vi "Stoerungen (385-448) - VFS4.vi"(8 "Fehler (Eingang)":errorcluster caption="Fehler (Eingang, kein Fehler)") -> (0 "Fehler (Ausgang)":errorcluster, 3 "Störungen 385-448":u64)   [LabVIEW 2015]
uses:
  PNS/Parameternamen PNS.ctl
  PNS/PNS.lvlib
  Stoerungen.lvlib
  Stoerungen Messgeraet/Aktionen Kommunikation Stoerung.ctl
  Seiten/System Einstellungen/System Einstellungen.lvlib
  Seiten/System Einstellungen/Aktioen FGV System.ctl
  PNS/Aktionen FGV Istwerte.ctl
  cRIO/Stoermeldungen/Stoerungen 385-448.ctl
  cRIO/Stoermeldungen/Stoermeldungen.lvlib
panel:
  # "Störmeldungen PNS (385-448)"
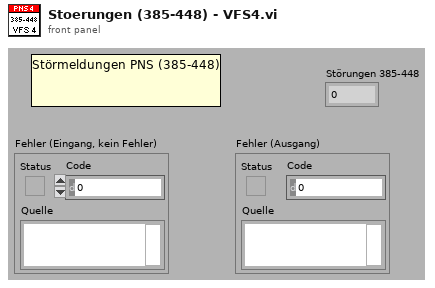
[diagram p1: front panel]
types:
  T1 = typedef "System Einstellungen.lvlib/Aktioen FGV System.ctl" = enum16{"lesen", "laden", "speichern", "Optionen schreiben", "Zeitstempel", "Reset BMP", "Reset SQP", "Wartung"}
  T2 = typedef "System Einstellungen.lvlib/Optionen.ctl" = cluster{"Störmeldep.":bool, "Betriebszustände":bool, "LN2 Befüllung":bool, "Klimaanlage ?":bool, "AK in ppm":bool, "log Cal-Gas":bool, "log 0-Gas":bool, "log CG zu PNS":bool, "Reserve":bool, "Reserve1":bool, "PNS?":bool, "Container":bool, "Mit N2 spülen":bool, "Span Gas Auswahl":T3, "VFS 1":bool, "VFS 2":bool, "VFS 3":bool, "VFS 4":bool, "TRE08":bool, "Leakcheck vor Kal":bool, "Amium 10-Fach":bool}
  T3 = typedef "Funktionstasten.lvlib/Spaneingang.ctl" = u16
  T4 = typedef "PNS.lvlib/Parameternamen PNS.ctl" = enum16{"Heizkreis 1", "Heizkreis 2", "Heizkreis 3", "Heizkreis 4", "Heizkreis 5", "Heizkreis 6", "Heizkreis 7", "Heizkreis 8"}
  T5 = typedef "PNS.lvlib/Aktionen FGV Istwerte.ctl" = enum16{"lesen", "initialisieren", "schreiben", "Störungen"}
  T6 = typedef "Stoerungen.lvlib/Aktionen Kommunikation Stoerung.ctl" = enum16{"lesen", "init", "FT-IR Komm", "FT-IR Betriebsart", "FT-IR Hintergrund", "cRIO Komm", "PNS Komm", "Dichtheitstest", "Life Bit", "FTIR Komm AK", "PMA Komm", "FID Komm", "PMA Cal", "FID Ch4 Cal", "FID THC Cal", "Cal Timeout", "VFS 1 Komm", "VFS 2 Komm", "VFS 3 Komm", "VFS 4 Komm", "TRE 08 Komm", "CG-Test vorzeitig", "CG-Test Span 1", "CG-Test Span 2", "CG-Test Span 3", "CG-Test Messgas", "CG-Test löschen", "Test", "Amium AK"}
  T7 = typedef "Stoermeldungen.lvlib/Stoerungen 385-448.ctl" = cluster{"ERR. 385":bool, "ERR. 386":bool, "ERR. 387":bool, "ERR. 388":bool, "ERR. 389":bool, "ERR. 390":bool, "ERR. 391":bool, "ERR. 392":bool, "ERR. 393":bool, "ERR. 394":bool, "ERR. 395":bool, "ERR. 396":bool, "ERR. 397":bool, "ERR. 398":bool, "ERR. 399":bool, "ERR. 400":bool, "ERR. 401":bool, "ERR. 402":bool, "ERR. 403":bool, "ERR. 404":bool, "ERR. 405":bool, "ERR. 406":bool, "ERR. 407":bool, "ERR. 408":bool, "ERR. 409":bool, "ERR. 410":bool, "ERR. 411":bool, "ERR. 412":bool, "ERR. 413":bool, "ERR. 414":bool, "ERR. 415":bool, "ERR. 416":bool, "ERR. 417":bool, "ERR. 418":bool, "ERR. 419":bool, "ERR. 420":bool, "ERR. 421":bool, "ERR. 422":bool, "ERR. 423":bool, "ERR. 424":bool, "ERR. 425":bool, "ERR. 426":bool, "ERR. 427":bool, "ERR. 428":bool, "ERR. 429":bool, "ERR. 430":bool, "ERR. 431":bool, "ERR. 432":bool, "ERR. 433":bool, "ERR. 434":bool, "ERR. 435":bool, "ERR. 436":bool, "ERR. 437":bool, "ERR. 438":bool, "ERR. 439":bool, "ERR. 440":bool, "ERR. 441":bool, "ERR. 442":bool, "ERR. 443":bool, "ERR. 444":bool, "ERR. 445":bool, "ERR. 446":bool, "ERR. 447":bool, "ERR. 448":bool}
  T8 = typedef "Steuerung PNS.lvclass/Regler.ctl" = cluster{"Istwert":i16, "Sollwert":i16, "Alarm MIN":i16, "Alarm MAX":i16, "Regler sperren":i16, "Analog Ausgang":i16}[]
  T9 = cluster{"Istwert":i16, "Sollwert":i16, "Alarm MIN":i16, "Alarm MAX":i16, "Regler sperren":i16, "Analog Ausgang":i16}
  T10 = typedef "Stoerungen.lvlib/Stoerungen Messgeraete.ctl" = cluster{"FT-IR Komm":bool, "FT-IR Betriebsart":bool, "FT-IR Hintergrundscan":bool, "Dichtheitstest":bool, "cRIO Komm":bool, "PNS Komm":bool, "Life Bit":bool, "FT-IR AK Komm":bool, "PMA Komm":bool, "FID Komm":bool, "PMA Cal":bool, "FID CH4 Cal":bool, "FID THC Cal":bool, "Cal Timeout":bool, "VFS 1 Komm":bool, "VFS 2 Komm":bool, "VFS 3 Komm":bool, "VFS 4 Komm":bool, "TRE 08 Komm":bool, "CG-Test":bool, "CG-Test 1":bool, "CG-Test 2":bool, "CG-Test 3":bool, "Messgas - Eingang":bool, "Amium AK Komm":bool}
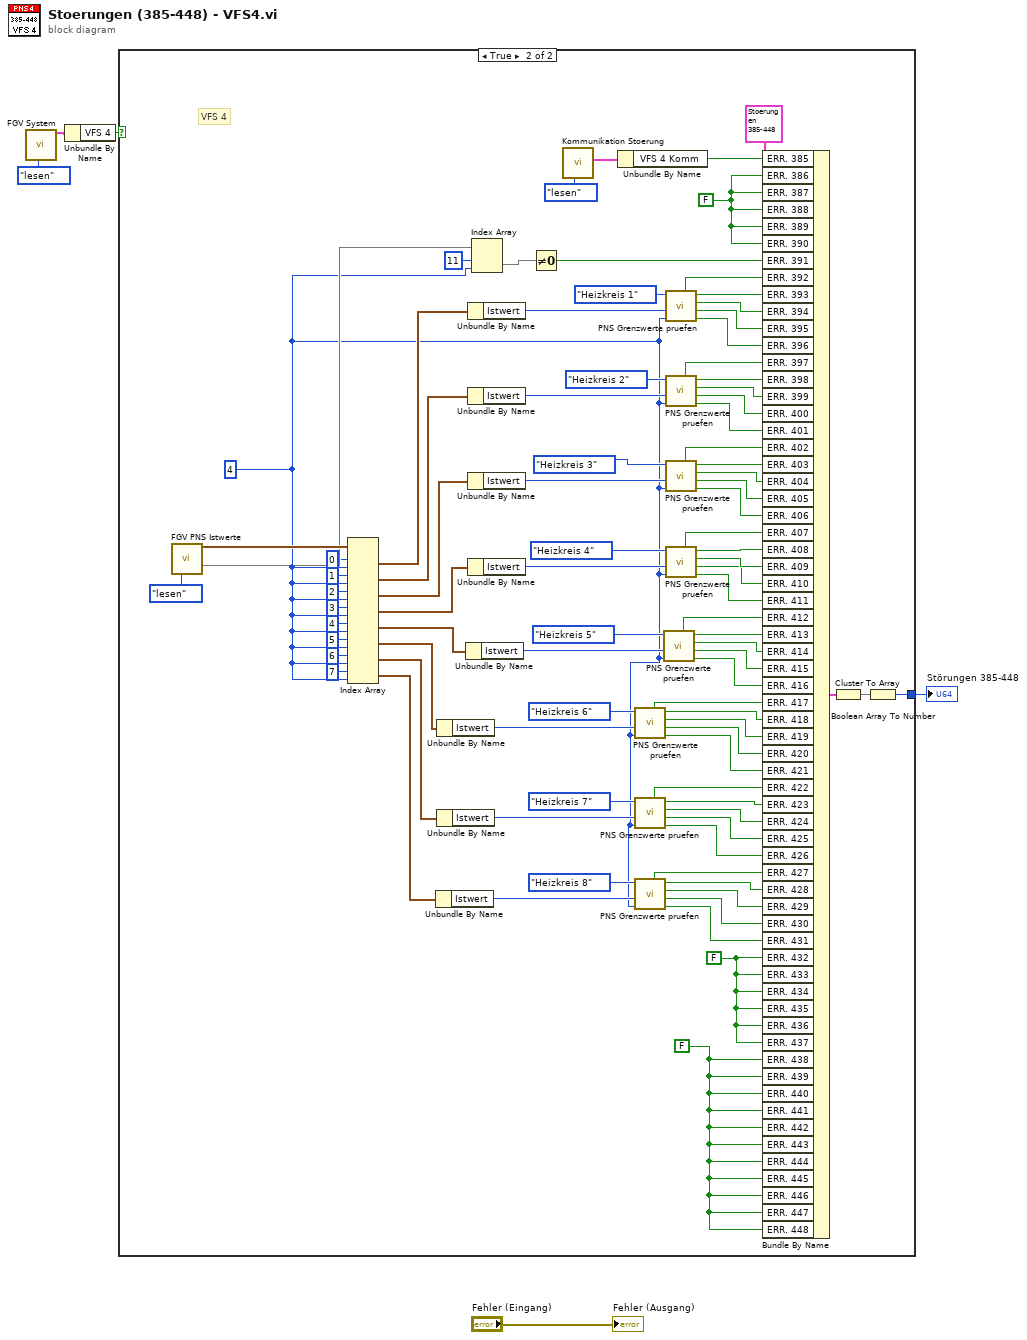
[diagram p0: block diagram]
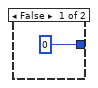
[diagram p2: hidden frame]
diagram:
  n1 = call "FGV System.vi"("Aktionen"=Aktioen_FGV_System."lesen") -> ("Optionen"=w3:T2)  [unwired: 13 in, 5 out]
  n2 = Unbundle By Name(w3) -> ("VFS 4"=w1:bool)
  n3 = case shown="True" w1 {
    tunnel: [u64 0 w55] -> w4
    frame False {
    }
    frame True {
      w7 = 4 ("Deaktivierter Index (Spalte)")
      w54 = FALSE ("ERR. 240")
      w62 = FALSE ("ERR. 194")
      w60 = FALSE ("ERR. 194")
      # "VFS 4"
      n4 = call "FGV PNS Istwerte.vi"("Aktionen"=Aktionen_FGV_Istwerte."lesen") -> ("Regler"=w92:T8, 10:w59)  [unwired: 10 in, 3 out]
      n5 = Index Array(array=w92, index (row) #1=0 ("Deaktivierter Index (Zeile)"), index (col) #1=w7, index (row) #2=1 ("Deaktivierter Index (Zeile)"), index (col) #2=w7, index (row) #3=2 ("Deaktivierter Index (Zeile)"), index (col) #3=w7, index (row) #4=3 ("Deaktivierter Index (Zeile)"), index (col) #4=w7, index (row) #5=4 ("Deaktivierter Index (Zeile)"), index (col) #5=w7, index (row) #6=5 ("Deaktivierter Index (Zeile)"), index (col) #6=w7, index (row) #7=6 ("Deaktivierter Index (Zeile)"), index (col) #7=w7, index (row) #8=7 ("Deaktivierter Index (Zeile)"), index (col) #8=w7) -> (element #1=w91:T9, element #2=w89:T9, element #3=w88:T9, element #4=w87:T9, element #5=w48:T9, element #6=w42:T9, element #7=w41:T9, element #8=w40:T9)
      n6 = Unbundle By Name(w40) -> ("Istwert"=w19:i16)
      n7 = Unbundle By Name(w42) -> ("Istwert"=w20:i16)
      n8 = Unbundle By Name(w41) -> ("Istwert"=w21:i16)
      n9 = Unbundle By Name(w48) -> ("Istwert"=w17:i16)
      n10 = Unbundle By Name(w91) -> ("Istwert"=w90:i16)
      n11 = Unbundle By Name(w89) -> ("Istwert"=w51:i16)
      n12 = Unbundle By Name(w88) -> ("Istwert"=w86:i16)
      n13 = Unbundle By Name(w87) -> ("Istwert"=w85:i16)
      n14 = Index Array(array=w59, index (row)=11 ("Index"), index (col)=w7) -> (element=w57)
      n15 = Not Equal To 0?(x=w57) -> (x != 0?=w56:bool)
      n16 = call "Kommunikation Stoerung.vi"("Aktionen"=Aktionen_Kommunikation_Stoerung."lesen") -> ("Störung Messgerät"=w64:T10)  [unwired: 10 in]
      n17 = Unbundle By Name(w64) -> ("VFS 4 Komm"=w61:bool)
      n18 = call "PNS Grenzwerte pruefen.vi"("Option"=w7, "Wert"=w20, "Parameternamen PNS"=Parameternamen_PNS."Heizkreis 6") -> ("AbschMax"=w35:bool, "AbschMin"=w36:bool, "WarnMax"=w37:bool, "WarnMin"=w38:bool, "F.Br."=w39:bool)  [unwired: 4 in]
      n19 = call "PNS Grenzwerte pruefen.vi"("Option"=w7, "Wert"=w21, "Parameternamen PNS"=Parameternamen_PNS."Heizkreis 7") -> ("AbschMax"=w30:bool, "AbschMin"=w31:bool, "WarnMax"=w32:bool, "WarnMin"=w33:bool, "F.Br."=w34:bool)  [unwired: 4 in]
      n20 = call "PNS Grenzwerte pruefen.vi"("Option"=w7, "Wert"=w19, "Parameternamen PNS"=Parameternamen_PNS."Heizkreis 8") -> ("AbschMax"=w25:bool, "AbschMin"=w26:bool, "WarnMax"=w27:bool, "WarnMin"=w28:bool, "F.Br."=w29:bool)  [unwired: 4 in]
      n21 = call "PNS Grenzwerte pruefen.vi"("Option"=w7, "Wert"=w17, "Parameternamen PNS"=Parameternamen_PNS."Heizkreis 5") -> ("AbschMax"=w43:bool, "AbschMin"=w44:bool, "WarnMax"=w45:bool, "WarnMin"=w46:bool, "F.Br."=w47:bool)  [unwired: 4 in]
      n22 = call "PNS Grenzwerte pruefen.vi"("Option"=w7, "Wert"=w90, "Parameternamen PNS"=Parameternamen_PNS."Heizkreis 1") -> ("AbschMax"=w80:bool, "AbschMin"=w81:bool, "WarnMax"=w82:bool, "WarnMin"=w83:bool, "F.Br."=w84:bool)  [unwired: 4 in]
      n23 = call "PNS Grenzwerte pruefen.vi"("Option"=w7, "Wert"=w51, "Parameternamen PNS"=Parameternamen_PNS."Heizkreis 2") -> ("AbschMax"=w75:bool, "AbschMin"=w76:bool, "WarnMax"=w77:bool, "WarnMin"=w78:bool, "F.Br."=w79:bool)  [unwired: 4 in]
      n24 = call "PNS Grenzwerte pruefen.vi"("Option"=w7, "Wert"=w86, "Parameternamen PNS"=Parameternamen_PNS."Heizkreis 3") -> ("AbschMax"=w70:bool, "AbschMin"=w71:bool, "WarnMax"=w72:bool, "WarnMin"=w73:bool, "F.Br."=w74:bool)  [unwired: 4 in]
      n25 = call "PNS Grenzwerte pruefen.vi"("Option"=w7, "Wert"=w85, "Parameternamen PNS"=Parameternamen_PNS."Heizkreis 4") -> ("AbschMax"=w65:bool, "AbschMin"=w66:bool, "WarnMax"=w67:bool, "WarnMin"=w68:bool, "F.Br."=w69:bool)  [unwired: 4 in]
      n26 = Bundle By Name(cluster=T7 {"ERR. 385"=FALSE, "ERR. 386"=FALSE, "ERR. 387"=FALSE, "ERR. 388"=FALSE, "ERR. 389"=FALSE, "ERR. 390"=FALSE, "ERR. 391"=FALSE, "ERR. 392"=FALSE, "ERR. 393"=FALSE, "ERR. 394"=FALSE, "ERR. 395"=FALSE, "ERR. 396"=FALSE, "ERR. 397"=FALSE, "ERR. 398"=FALSE, "ERR. 399"=FALSE, "ERR. 400"=FALSE, "ERR. 401"=FALSE, "ERR. 402"=FALSE, "ERR. 403"=FALSE, "ERR. 404"=FALSE, "ERR. 405"=FALSE, "ERR. 406"=FALSE, "ERR. 407"=FALSE, "ERR. 408"=FALSE, "ERR. 409"=FALSE, "ERR. 410"=FALSE, "ERR. 411"=FALSE, "ERR. 412"=FALSE, "ERR. 413"=FALSE, "ERR. 414"=FALSE, "ERR. 415"=FALSE, "ERR. 416"=FALSE, "ERR. 417"=FALSE, "ERR. 418"=FALSE, "ERR. 419"=FALSE, "ERR. 420"=FALSE, "ERR. 421"=FALSE, "ERR. 422"=FALSE, "ERR. 423"=FALSE, "ERR. 424"=FALSE, "ERR. 425"=FALSE, "ERR. 426"=FALSE, "ERR. 427"=FALSE, "ERR. 428"=FALSE, "ERR. 429"=FALSE, "ERR. 430"=FALSE, "ERR. 431"=FALSE, "ERR. 432"=FALSE, "ERR. 433"=FALSE, "ERR. 434"=FALSE, "ERR. 435"=FALSE, "ERR. 436"=FALSE, "ERR. 437"=FALSE, "ERR. 438"=FALSE, "ERR. 439"=FALSE, "ERR. 440"=FALSE, "ERR. 441"=FALSE, "ERR. 442"=FALSE, "ERR. 443"=FALSE, "ERR. 444"=FALSE, "ERR. 445"=FALSE, "ERR. 446"=FALSE, "ERR. 447"=FALSE, "ERR. 448"=FALSE} ("STÖRUNGEN 193-256"), "ERR. 385"=w61, "ERR. 386"=w60, "ERR. 387"=w60, "ERR. 388"=w60, "ERR. 389"=w60, "ERR. 390"=w60, "ERR. 391"=w56, "ERR. 392"=w84, "ERR. 393"=w83, "ERR. 394"=w82, "ERR. 395"=w81, "ERR. 396"=w80, "ERR. 397"=w79, "ERR. 398"=w78, "ERR. 399"=w77, "ERR. 400"=w76, "ERR. 401"=w75, "ERR. 402"=w74, "ERR. 403"=w73, "ERR. 404"=w72, "ERR. 405"=w71, "ERR. 406"=w70, "ERR. 407"=w69, "ERR. 408"=w68, "ERR. 409"=w67, "ERR. 410"=w66, "ERR. 411"=w65, "ERR. 412"=w47, "ERR. 413"=w46, "ERR. 414"=w45, "ERR. 415"=w44, "ERR. 416"=w43, "ERR. 417"=w39, "ERR. 418"=w38, "ERR. 419"=w37, "ERR. 420"=w36, "ERR. 421"=w35, "ERR. 422"=w34, "ERR. 423"=w33, "ERR. 424"=w32, "ERR. 425"=w31, "ERR. 426"=w30, "ERR. 427"=w29, "ERR. 428"=w28, "ERR. 429"=w27, "ERR. 430"=w26, "ERR. 431"=w25, "ERR. 432"=w54, "ERR. 433"=w54, "ERR. 434"=w54, "ERR. 435"=w54, "ERR. 436"=w54, "ERR. 437"=w54, "ERR. 438"=w62, "ERR. 439"=w62, "ERR. 440"=w62, "ERR. 441"=w62, "ERR. 442"=w62, "ERR. 443"=w62, "ERR. 444"=w62, "ERR. 445"=w62, "ERR. 446"=w62, "ERR. 447"=w62, "ERR. 448"=w62) -> (w95:T7)
      n27 = Cluster To Array(cluster=w95) -> (array=w94:bool[])
      n28 = Boolean Array To Number ("Boolesches Array nach Zahl")(Boolean array=w94) -> (number=w55:u64)
    }
  }
  "Störungen 385-448" <- w4
  "Fehler (Ausgang)" <- "Fehler (Eingang)"
